vi "CLD 11 Producer consumer events front panel.vi"() -> ()   [LabVIEW 2009]
doc: "CLD 11 exercise"
panel:
  out "Current Time target":dbl
  out "Step 3":bool
  out "Step 2":bool
  out "Step 1":bool
  out "Time Has Elapsed":bool
  out "Elapsed Time":string
  in  "Auto Reset":bool
  in  "Reset Button":bool
  in  "Stop VI":bool
  in  "Time Target (s)":dbl
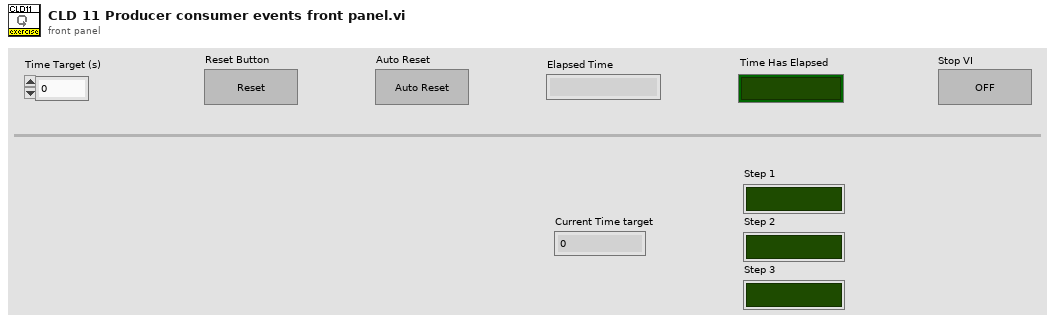
[diagram p1: front panel]
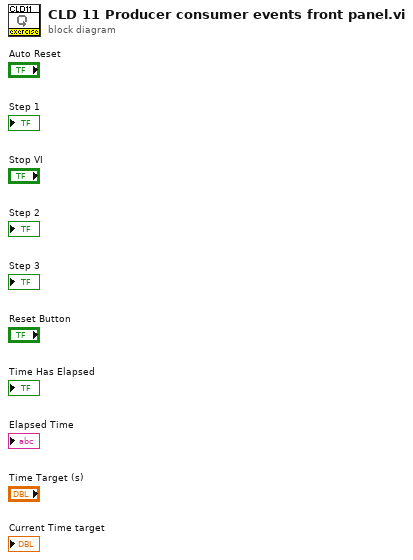
[diagram p0: block diagram]
diagram:
